vi "GenericStatusIndicator.vi"(9 "Total":i32, 10 "Current Iteration":i32) -> (3 "Status":string)   [LabVIEW 2023, in "CICD.lvlib"]
uses:
  CICD.lvlib
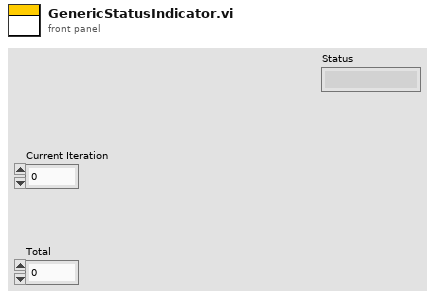
[diagram p1: front panel]
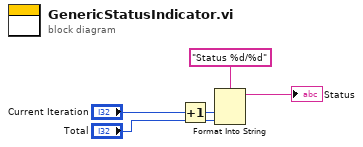
[diagram p0: block diagram]
diagram:
  n1 = Increment(x="Current Iteration") -> (x+1=w1:i32)
  n2 = Format Into String(format string="Status %d/%d", w1, "Total") -> (resulting string=→"Status":string)  [unwired: 2 in, 1 out]
